vi "DS402-manager-Main.vi"() -> ()   [LabVIEW 2016]
uses:
  NationalInstruments.VeriStand.SystemStorageUI
  NationalInstruments.VeriStand.SystemStorage
  <vilib>/NI Veristand/Templates/Workspace Tool Support/Workspace Tool Message Bus.ctl
  <vilib>/NI Veristand/Templates/Workspace Tool Support/Workspace Tool Message (String).ctl
  <vilib>/NI Veristand/Templates/Workspace Tool Support/Workspace Tool Response (String).ctl
  <vilib>/NI Veristand/Templates/Workspace Tool Support/Workspace Tool Message (Byte Array).ctl
  <vilib>/NI Veristand/Templates/Workspace Tool Support/Workspace Tool Response (Byte Array).ctl
  _qmh/controls/UI Data.ctl
  _qmh/support/Message Queue/Enqueue Message (Single).vi
  <vilib>/Utility/error.llb/Error Cluster From Error Code.vi
  <vilib>/NI Veristand/Execution/Workspace/NI VeriStand - Get Multiple Channel Values.vi
  <vilib>/ErrorRing/Error Ring.xnode
  <vilib>/NI VeriStand/Execution/Workspace/NI_VS Workspace ExecutionAPI.lvlib
  <vilib>/NI Veristand/UI Controls/System Definition Tree/NI_VS UI System Tree.lvlib
  ds402mgr_Helper/ds402mgr_Helper.lvlib
  _qmh/support/User Event - Stop/User Event - Stop.lvlib
  _qmh/support/Message Queue/Message Queue.lvlib
  <vilib>/NI VeriStand/Templates/Workspace Tool Support/NI VeriStand - Workspace Tool Support.lvlib
panel:
  in  "Targets":i32(listbox)
  out "Detected at":timestamp
  out "Error":bool
  out "Slave Transition State history":string
  out "Slave State - Current":string
  in  "Tab Control":enum32{"Debug", "SDO", "Slave Diagnostics"}(tab)
  out "names":string[](array[string])
  out "types":i32[](array[ring]) items=["K_STRING", "K_BOOL", "K_I32", "K_U32", "K_DOUBLE", "K_U64", "K_VARIANT", "K_DEPENDENTFILE", "K_DEPENDENTNODE", "K_DATASOURCENODE", "K_U16", "K_DBLARR", "K_U32ARR", "K_I32ARR", "K_STRINGARR", "K_DICTIONARY", "K_DICTIONARYARR", "K_BINARYSTRING", "K_I16", "K_I64", "K_BOOLARR", "K_U64ARR", "K_U16ARR", "K_I64ARR", "K_I16ARR"]
  in  "width":enum16{"U8", "U16", "U32"}(ring)
  in  "Value to Write":i32
  out "Value Read":i32
  in  "Blocking Write":bool=TRUE
  in  "Abort Write":bool
  in  "Do Action":bool
  in  "Action":enum16{"Read", "Write"}(ring)
  out "Raw Data Read":u8[](array[numeric]) format="%.0x"
  out "Raw  - Data to Write":u8[](array[numeric]) format="%.0x"
  in  "Cleare Errors":bool
  out "Error Ext Para":i32[](array[numeric]) format="%.0x"
  out "Error Ext":u32
  out "Last Error":i32 format="%.0x"
  out "Abort Code":u32 format="%.0x"
  out "EMCY Data":T1 {"Error Code" format="%.0x"}
  out "Error Out":errorcluster
  in  "Action 4":bool
  in  "Action 3":bool
  in  "Action 2":bool
  in  "Action 1":bool
  out "Slave Information":string
  in  "NIVS.Message Bus":T2
  in  "Stop":bool
  in  "NIVS.System Definition Root":refnum<k24>
  in  "Select EtherCAT Slave":refnum<k24>(container)
  in  "NIVS.Project File Path":path
  in  "NIVS.Workspace Event":refnum<event-registration>
  out "System Times":dbl[](array[numeric]) format="%<%H:%M:%S%3u>t"
  out "Targets":string[](array[string])
  in  "NIVS.Gateway IP Address":string
  in  "NIVS.INI File Path":path
  # "With the assistance of the NI VeriStand Execution API, a tool has access to streaming data running on the target."
  # "This is the file path to the VeriStand system definition file. You can read or write to the file using the System Definition API."
  # "This is the root reference to the active System Definition file. You could use this to read the configuration or populate a tree with channels. You are free to close this reference, but it will be closed for you if you don't."
  # "This is the IP Address of the VeriStand Gateway to which the Workspace is connected. Use this to open all the .NET Manager references. Usually the Gateway is running on localhost, but it could be running on a neighbor's machine."
  # "This registered string User Event is used to help instruct your tool to shut down when the Workspace is closing."
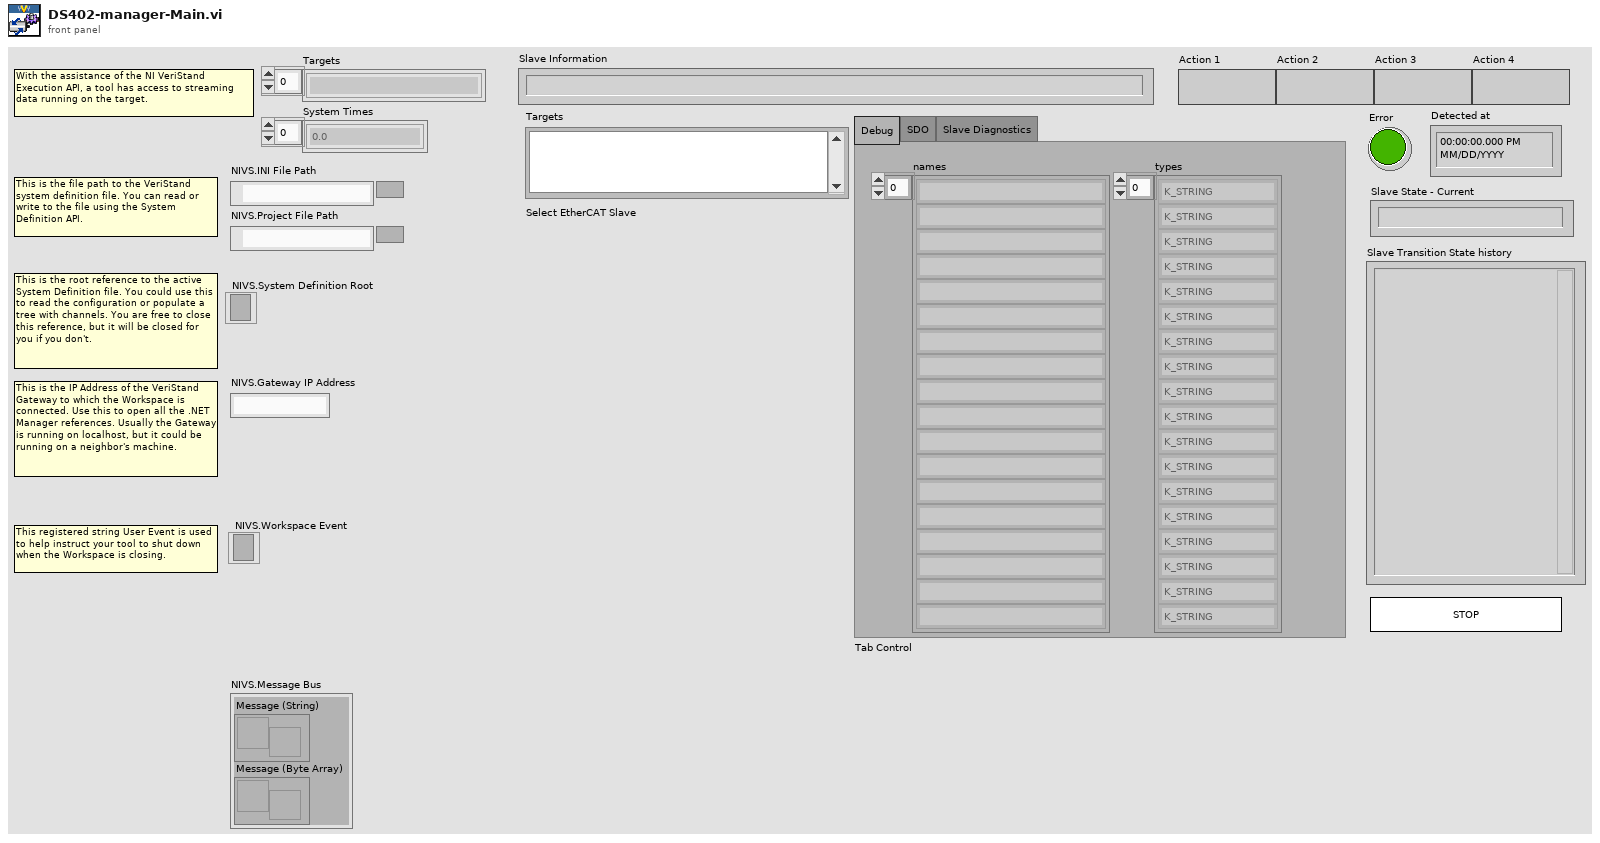
[diagram p1: front panel]
types:
  T1 = cluster{"Emergency Data":dbl[], "Error Register":u8, "Error Code":u16}
  T2 = typedef "NI VeriStand - Workspace Tool Support.lvlib/Workspace Tool Message Bus.ctl" = cluster{"Message (String)":refnum<user-event>, "Message (Byte Array)":refnum<user-event>}
  T3 = typedef "UI Data.ctl" = cluster{"Boolean <Replace Me>":bool, "String <Replace Me>":string, "Numeric <Replace Me>":dbl, "Do Something Ref":refnum<vi>, "Do Something Else Ref":refnum<vi>, "Data Display Ref":refnum<vi>, "Exit Button Ref":refnum<vi>}
  T4 = typedef "NI_VS Workspace ExecutionAPI.lvlib/WorkspaceAPI.ctl" = refnum<k24>
  T5 = typedef "ds402mgr_Helper.lvlib/_targetDetails.ctl" = cluster{"IP address":string, "NodeRef":refnum<k24>}
  T6 = typedef "NI_VS UI System Tree.lvlib/Callback Type.ctl" = cluster{"Net Callbacks":refnum<k27>[], "Event":T7}
  T7 = typedef "NI_VS UI System Tree.lvlib/Net Event Data Ref.ctl" = refnum<user-event>
  T8 = typedef "Message Queue.lvlib/All Message Queues.ctl" = cluster{"UI":refnum<queue>}
  T9 = typedef "NI_VS Workspace ExecutionAPI.lvlib/SystemStateEventRef.ctl" = cluster{"CustDatRef":refnum<user-event>, "EvtRef":refnum<k27>, "Target State User Event":refnum<user-event>}
  T10 = typedef "NI_VS Workspace ExecutionAPI.lvlib/SystemStateRegEventRef.ctl" = refnum<event-registration>
  T11 = cluster{"Event Registration Refnum":refnum<event-registration>, "NIVS.Workspace Event":refnum<event-registration>, "SystemChangeEventRef":T10}
  T12 = typedef "NI_VS UI System Tree.lvlib/Node Ref.ctl" = refnum<k24>
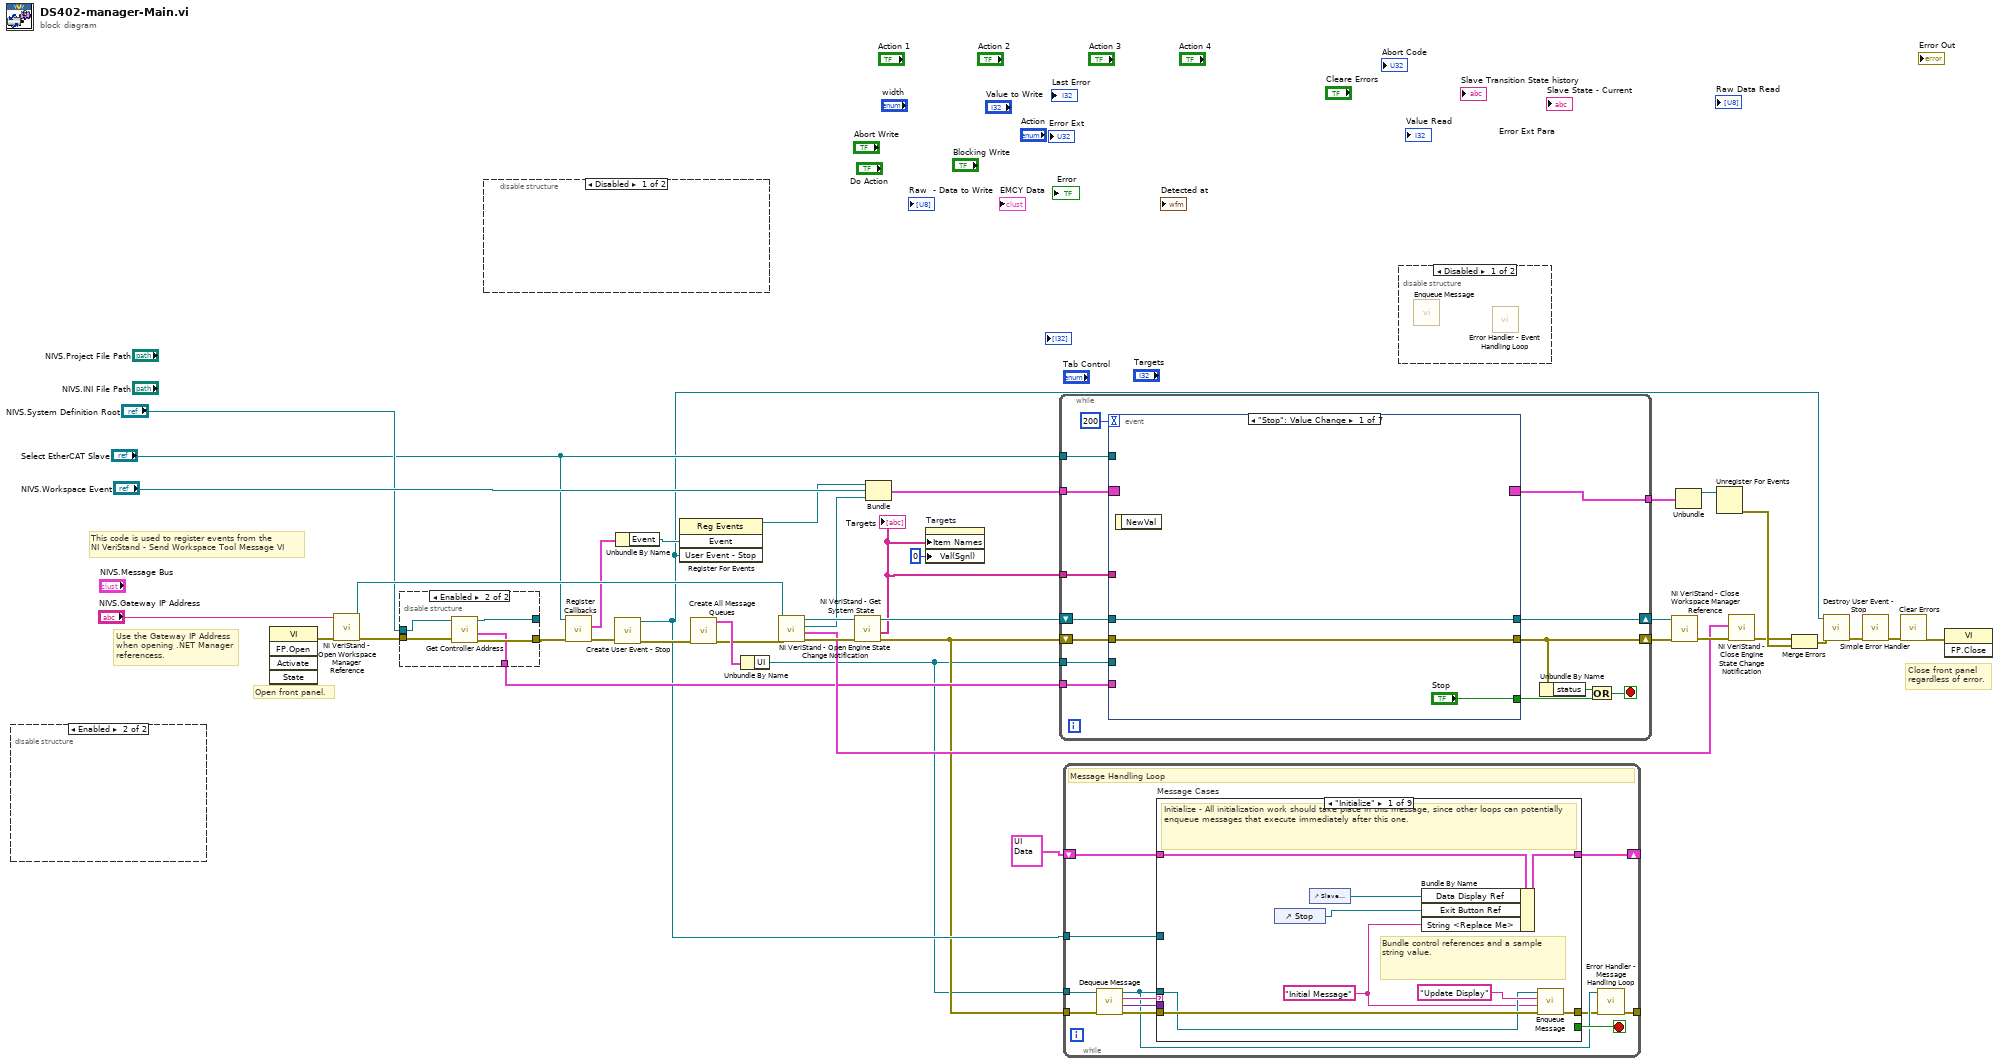
[diagram p0: block diagram]
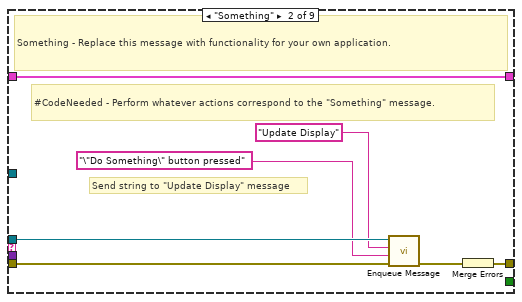
[diagram p3: hidden frame]
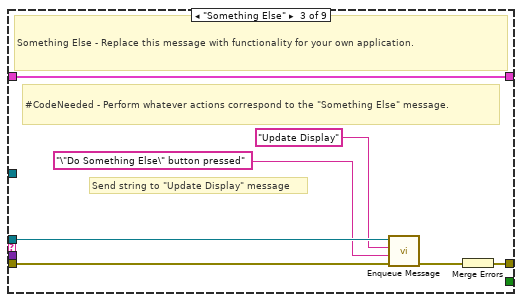
[diagram p4: hidden frame]
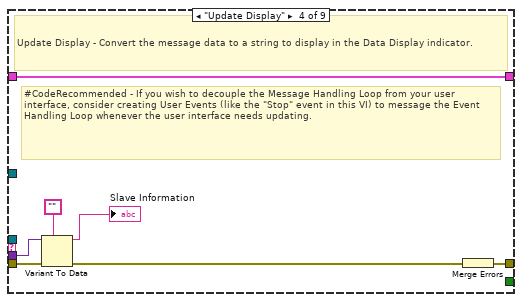
[diagram p5: hidden frame]
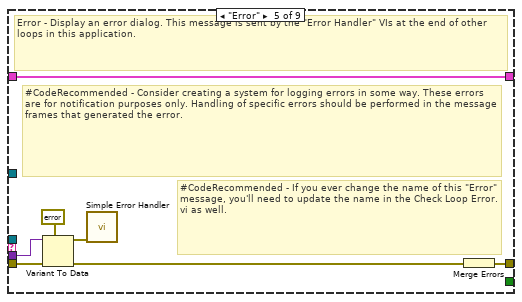
[diagram p6: hidden frame]
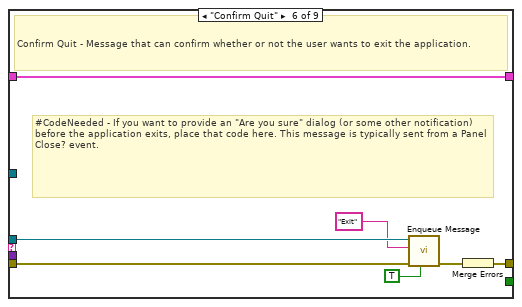
[diagram p7: hidden frame]
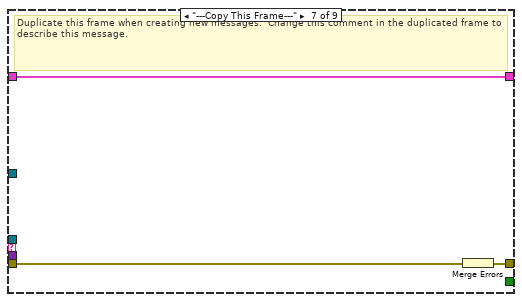
[diagram p8: hidden frame]
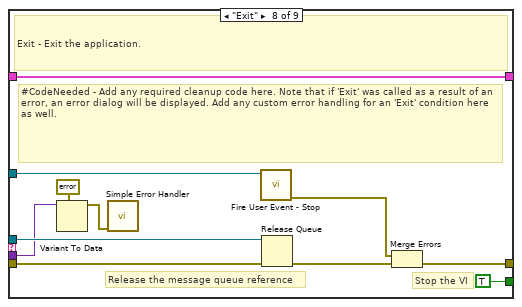
[diagram p9: hidden frame]
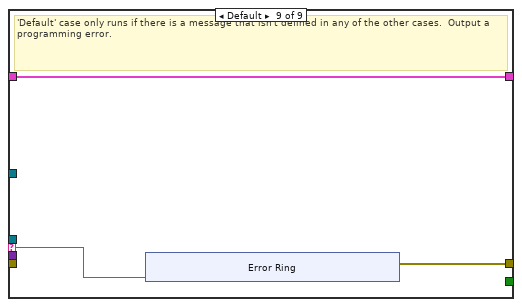
[diagram p10: hidden frame]
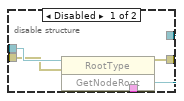
[diagram p12: hidden frame]
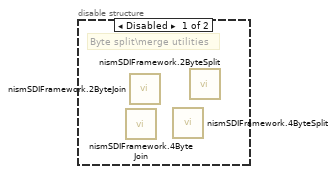
[diagram p13: hidden frame]
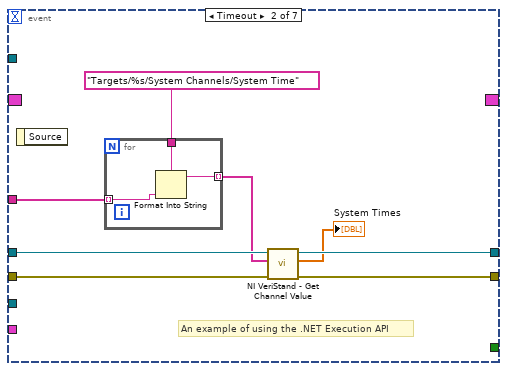
[diagram p14: hidden frame]
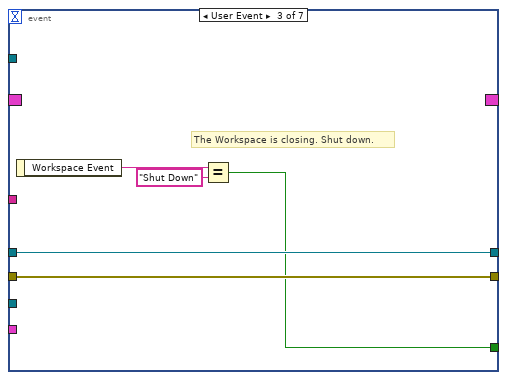
[diagram p15: hidden frame]
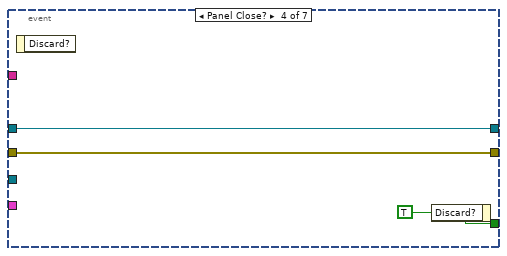
[diagram p16: hidden frame]
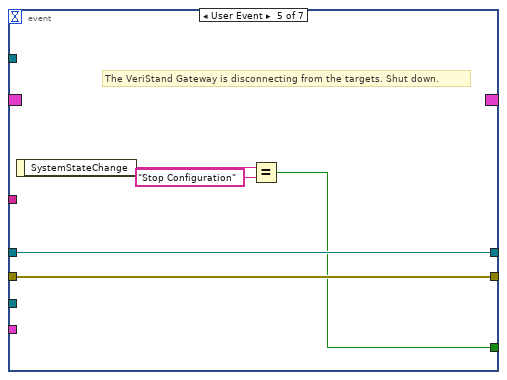
[diagram p17: hidden frame]
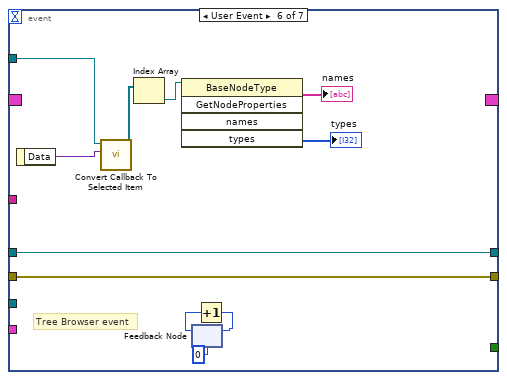
[diagram p18: hidden frame]
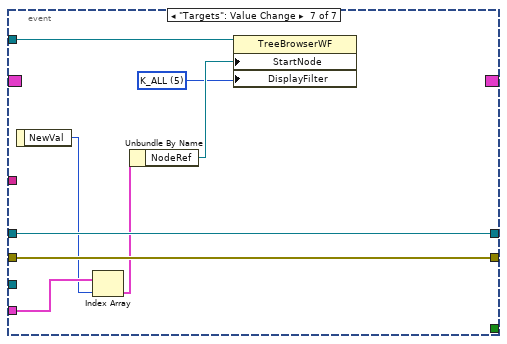
[diagram p19: hidden frame]
diagram:
  # "This code is used to register events from the\nNI VeriStand - Send Workspace Tool Message VI"
  # "Use the Gateway IP Address when opening .NET Manager referencess."
  # "Close front panel\nregardless of error."
  # "Open front panel."
  n1 = disable-structure shown="Enabled" {
    frame Disabled {
      # "Byte split\\merge utilities"
      n2 = call <vilib>:"nismSDIFramework.4ByteJoin.vi"() -> ()  [unwired: 11 in, 1 out]
      n3 = call <vilib>:"nismSDIFramework.2ByteJoin.vi"() -> ()  [unwired: 11 in, 1 out]
      n4 = call <vilib>:"nismSDIFramework.4ByteSplit.vi"() -> ()  [unwired: 8 in, 4 out]
      n5 = call <vilib>:"nismSDIFramework.2ByteSplit.vi"() -> ()  [unwired: 10 in, 2 out]
    }
    frame Enabled {
    }
  }
  n6 = invoke class="VI" method="FP.Open"() -> (error out=w26:errorcluster)  [unwired: 5 in, 4 out]
  n7 = call <vilib>:"NI VeriStand - Open Workspace Manager Reference.vi"("error in (no error)"=w26, "Gateway IP Address (\"\": localhost)"="NIVS.Gateway IP Address") -> ("error out"=w17:errorcluster, "WorkspaceManager"=w34:T4)  [unwired: 8 in]
  n8 = disable-structure shown="Enabled" {
    disable-tunnel: [w43 w46] -> _
    disable-tunnel: [w42 w47] -> w16
    disable-tunnel: "NIVS.System Definition Root" -> [w41 w48]
    disable-tunnel: w17 -> [w40 w45]
    disable-tunnel: [_ w44] -> w15
    frame Disabled {
      n9 = invoke class="RootType" method="GetNodeRoot"(reference=w41, error in=w40) -> (error out=w42:errorcluster, "GetNodeRoot"=w43:refnum<k24>)  [unwired: 1 in, 1 out]
    }
    frame Enabled {
      n10 = call "Get Controller Address.vi"("error in (no error)"=w45, "NIVS.System Definition Root In"=w48) -> ("error out"=w47:errorcluster, "Results"=w44:T5[], "NIVS.System Definition Root Out"=w46:refnum<k24>)  [unwired: 5 in, 2 out]
    }
  }
  n11 = disable-structure shown="Disabled" {
    frame Disabled {
    }
    frame Enabled {
    }
  }
  n12 = call <vilib>:"Register Callbacks.vi"("error in (no error)"=w16, "System Definition Tree"="Select EtherCAT Slave") -> ("error out"=w12:errorcluster, "Callbacks"=w20:T6)  [unwired: 7 in, 1 out]
  n13 = call "Create User Event - Stop.vi"("error in (no error)"=w12) -> ("error out"=w10:errorcluster, "User Event - Stop"=w3:refnum<user-event>)  [unwired: 9 in]
  n14 = Unbundle By Name(w20) -> ("Event"=w19:T7)
  n15 = register-events(w19, w3) -> (reference out=w18:refnum<event-registration>)  [unwired: 2 in, 1 out]
  n16 = call "Create All Message Queues.vi"("error in (no error)"=w10) -> ("error out"=w9:errorcluster, "Message Queues out"=w11:T8)  [unwired: 9 in]
  n17 = Unbundle By Name(w11) -> ("UI"=w1:refnum<queue>)
  n18 = call <vilib>:"NI VeriStand - Open Engine State Change Notification.vi"("error in (no error)"=w9, "WorkspaceManager in"=w34) -> ("error out"=w38:errorcluster, "SystemStateRefs"=w29:T9, "SystemChangeEventRef"=w23:T10, "WorkspaceManager out"=w39:T4)  [unwired: 6 in]
  n19 = call <vilib>:"NI VeriStand - Get System State.vi"("error in (no error)"=w38, "WorkspaceManager in"=w39) -> ("error out"=w2:errorcluster, "Targets"=w14:string[], "WorkspaceManager  out"=w28:T4)  [unwired: 5 in, 2 out]
  "Targets" <- w14
  n20 = Bundle("Event Registration Refnum"=w18, "NIVS.Workspace Event"="NIVS.Workspace Event", "SystemChangeEventRef"=w23) -> (w33:T11)  [unwired: 1 in]
  n21 = property on="Targets" class="LstBox (strict)"("Item Names"=w14, "Val(Sgnl)"=0 ("Value (Signaling)")) -> ()  [unwired: 2 in, 2 out]
  n22 = while {
    tunnel: w33 -> [w62]
    tunnel: [w61] -> w32
    shift-right: [w55] -> w35
    shift-left: w2 -> [w59]
    shift-right: [w58] -> w36
    shift-left: w28 -> [w60]
    tunnel: "Select EtherCAT Slave" -> [w52]
    tunnel: w15 -> [w51]
    tunnel: w14 -> [w50]
    tunnel: w1 -> [w49]
    stop <- w53 stop-if-true
    n23 = event shown="[0] \"Stop\": Value Change" {
      selector: w62 -> [_ _ _ _ _ _ _]
      dyn-events: [_ _ _ _ _ _ _] -> w61
      timeout: 200 -> [_ _ _ _ _ _ _]
      tunnel: ["Stop" _ w77 w82 w85 _ _] -> w54
      tunnel: w60 -> [w64 w73 w80 w83 w88 w99 w107]
      tunnel: w59 -> [w65 w72 w81 w84 w89 w100 w108]
      tunnel: [w65 w68 w81 w84 w89 w100 w108] -> w55
      tunnel: [w64 w69 w80 w83 w88 w99 w107] -> w58
      tunnel: w52 -> [_ _ _ _ _ w95 w104]
      tunnel: w51 -> [_ _ _ _ _ _ w106]
      tunnel: w50 -> [_ w66 _ _ _ _ _]
      tunnel: w49 -> [_ _ _ _ _ _ _]
      event "Stop": Value Change {
        n24 = event-data() -> ()  [unwired: 1 in, 1 out]
      }
      event Timeout {
        # "An example of using the .NET Execution API"
        n25 = event-data() -> ()  [unwired: 1 in, 1 out]
        n26 = for {
          tunnel: "Targets/%s/System Channels/System Time" ("format string") -> [w76]
          tunnel: [w75] -> w70 mode=indexing
          tunnel: w66 -> [w74] mode=indexing
          n27 = Format Into String(format string=w76, w74) -> (resulting string=w75:string)  [unwired: 2 in, 1 out]
        }
        n28 = call-poly <vilib>:"NI VeriStand - Get Channel Value.vi"("error in (no error)"=w72, "Channels"=w70, "WorkspaceManager in"=w73) -> ("error out"=w68:errorcluster, "Values"=→"System Times":dbl[], "WorkspaceManager out"=w69:T4)  [unwired: 6 in]
      }
      event User Event {
        # "The Workspace is closing. Shut down."
        n29 = event-data() -> ("Workspace Event"=w79:string)  [unwired: 1 in]
        n30 = Equal?(x=w79, y="Shut Down") -> (x = y?=w77:bool)
      }
      event Panel Close? {
        w82 = TRUE ("Discard?")
        n31 = event-data() -> ()  [unwired: 1 in, 1 out]
        n32 = event-data("Discard?"=w82) -> ()  [unwired: 1 in, 1 out]
      }
      event User Event {
        # "The VeriStand Gateway is disconnecting from the targets. Shut down."
        n33 = event-data() -> ("SystemStateChange"=w87:string)  [unwired: 1 in]
        n34 = Equal?(x=w87, y="Stop Configuration") -> (x = y?=w85:bool)
      }
      event User Event {
        # "Tree Browser event"
        n35 = event-data() -> ("Data"=w96:variant)  [unwired: 1 in]
        n36 = call <vilib>:"Convert Callback To Selected Item.vi"("Data"=w96, "SystemDefinitionBrowser Ref"=w95) -> ("Selected Item"=w93:T12[])  [unwired: 8 in, 1 out]
        n37 = Index Array(array=w93) -> (element=w91:T12)  [unwired: 1 in]
        n38 = invoke class="BaseNodeType" method="GetNodeProperties"(reference=w91) -> ("names"=→"names":string[], "types"=→"types":i32[])  [unwired: 4 in, 3 out]
        n39 = feedback #1(0) -> (w90:i32)
        n40 = Increment(x=w90) -> (x+1=w98:i32)
        n41 = feedback-in #1(w98) -> ()
      }
      event "Targets": Value Change {
        w101 = u8 5 items=["K_CHAN_R", "K_CHAN_W", "K_CHAN_RW", "K_CHAN_VOLT", "K_CHAN_FAULT", "K_ALL", "K_CUSTOM", "K_CHAN_R_VIS", "K_CHAN_W_VIS", "K_CHAN_RW_VIS", "K_CHAN_VOLT_VIS", "K_CHAN_FAULT_VIS"] ("DisplayFilter")
        n42 = event-data() -> ("NewVal"=w105:i32)  [unwired: 1 in]
        n43 = Index Array(array=w106, index=w105) -> (element=w103:T5)
        n44 = Unbundle By Name(w103) -> ("NodeRef"=w102:refnum<k24>)
        n45 = property class="TreeBrowserWF"(reference=w104, "StartNode"=w102, "DisplayFilter"=w101) -> ()  [unwired: 1 in, 2 out]
      }
    }
    n46 = Unbundle By Name(w55) -> ("status"=w56:bool)
    n47 = Compound Arithmetic op=OR(w56, w54) -> (w53:bool)
  }
  n48 = while {
    tunnel: w1 -> [w112]
    shift-right: [w119] -> _
    shift-left: T3 {"Boolean <Replace Me>"=FALSE, "String <Replace Me>"="", "Numeric <Replace Me>"=0.0, "Do Something Ref"=refnum, "Do Something Else Ref"=refnum, "Data Display Ref"=refnum, "Exit Button Ref"=refnum} ("Data Cluster") -> [w120]
    tunnel: w3 -> [w117]
    tunnel: w2 -> [w116]
    tunnel: [w110] -> _
    stop <- w118 stop-if-true
    # "Message Handling Loop"
    n49 = call "Dequeue Message.vi"("error in (no error)"=w116, "Message Queue"=w112) -> ("error out"=w115:errorcluster, "Message Data"=w113:variant, "Message"=w114:string, "dup Message Queue"=w111:refnum<queue>)  [unwired: 6 in]
    n50 = case "Message Cases" shown="\"Initialize\"" w114 {
      selector: w114 -> [_ _ _ _ _ _ _ _ w179]
      tunnel: w111 -> [w124 w132 w139 _ _ w160 _ w178 _]
      tunnel: w115 -> [w128 w134 w141 w148 w157 w164 w167 w171 _]
      tunnel: [w129 w135 w142 w149 w151 w162 w165 w174 w180] -> w109
      tunnel: w120 -> [w127 w136 w143 w150 w156 w163 w166 w177 w181]
      tunnel: [w126 w136 w143 w150 w156 w163 w166 w177 w181] -> w119
      tunnel: [_ _ _ _ _ _ _ TRUE _] -> w118
      tunnel: w113 -> [_ _ _ w147 w155 _ _ w168 _]
      tunnel: w117 -> [_ _ _ _ _ _ _ w173 _]
      frame "Initialize" {
        w123 = "Initial Message" ("Initial Message")
        # "Bundle control references and a sample string value."
        # "Initialize - All initialization work should take place in this message, since other loops can potentially enqueue messages that execute immediately after this one."
        n51 = control-ref of="Stop"() -> (w121:refnum<vi>)
        n52 = control-ref of="Slave Information"() -> (w122:refnum<vi>)
        n53 = Bundle By Name(cluster=w127, "Data Display Ref"=w122, "Exit Button Ref"=w121, "String <Replace Me>"=w123) -> (w126:T3)
        n54 = call-poly "Enqueue Message.vi"("error in (no error)"=w128, "Message Data"=w123, "Message"="Update Display", "Message Queue"=w124) -> ("error out"=w129:errorcluster)  [unwired: 6 in, 1 out]
      }
      frame "Something" {
        # "Send string to \"Update Display\" message"
        # "#CodeNeeded - Perform whatever actions correspond to the \"Something\" message."
        # "Something - Replace this message with functionality for your own application."
        n55 = call-poly "Enqueue Message.vi"("error in (no error)"=w134, "Message Data"="\"Do Something\" button pressed" ("\"Do Something\" button pressed"), "Message"="Update Display", "Message Queue"=w132) -> ("error out"=w133:errorcluster)  [unwired: 6 in, 1 out]
        n56 = Merge Errors(w133) -> (w135:errorcluster)
      }
      frame "Something Else" {
        # "Send string to \"Update Display\" message"
        # "#CodeNeeded - Perform whatever actions correspond to the \"Something Else\" message."
        # "Something Else - Replace this message with functionality for your own application."
        n57 = call-poly "Enqueue Message.vi"("error in (no error)"=w141, "Message Data"="\"Do Something Else\" button pressed" ("\"Do Something Else\" button pressed"), "Message"="Update Display", "Message Queue"=w139) -> ("error out"=w140:errorcluster)  [unwired: 6 in, 1 out]
        n58 = Merge Errors(w140) -> (w142:errorcluster)
      }
      frame "Update Display" {
        # "#CodeRecommended - If you wish to decouple the Message Handling Loop from your user interface, consider creating User Events (like the \"Stop\" event in this VI) to message the Event Handling Loop whenever the user interface needs updating."
        # "Update Display - Convert the message data to a string to display in the Data Display indicator."
        n59 = Variant To Data(error in=w148, type="", Variant=w147) -> (data=→"Slave Information":string, error out=w145:errorcluster)
        n60 = Merge Errors(w145) -> (w149:errorcluster)
      }
      frame "Error" {
        # "#CodeRecommended - If you ever change the name of this \"Error\" message, you'll need to update the name in the Check Loop Error.vi as well."
        # "#CodeRecommended - Consider creating a system for logging errors in some way. These errors are for notification purposes only. Handling of specific errors should be performed in the message frames that generated the error."
        # "Error - Display an error dialog. This message is sent by the \"Error Handler\" VIs at the end of other loops in this application."
        n61 = Variant To Data(error in=w157, type=errorcluster {"status"=FALSE, "code"=0, "source"=""} ("error constant"), Variant=w155) -> (data=w153:errorcluster, error out=w152:errorcluster)
        n62 = call <vilib>:"Simple Error Handler.vi"("error in (no error)"=w153) -> ()  [unwired: 4 in, 5 out]
        n63 = Merge Errors(w152) -> (w151:errorcluster)
      }
      frame "Confirm Quit" {
        # "#CodeNeeded - If you want to provide an \"Are you sure\" dialog (or some other notification) before the application exits, place that code here. This message is typically sent from a Panel Close? event."
        # "Confirm Quit - Message that can confirm whether or not the user wants to exit the application."
        n64 = call-poly "Enqueue Message.vi"("Priority Message? (F)"=TRUE, "error in (no error)"=w164, "Message"="Exit", "Message Queue"=w160) -> ("error out"=w161:errorcluster)  [unwired: 6 in, 1 out]
        n65 = Merge Errors(w161) -> (w162:errorcluster)
      }
      frame "---Copy This Frame---" {
        # "Duplicate this frame when creating new messages.  Change this comment in the duplicated frame to describe this message."
        n66 = Merge Errors(w167) -> (w165:errorcluster)
      }
      frame "Exit" {
        # "Stop the VI"
        # "Release the message queue reference"
        # "#CodeNeeded - Add any required cleanup code here. Note that if 'Exit' was called as a result of an error, an error dialog will be displayed. Add any custom error handling for an 'Exit' condition here as well."
        # "Exit - Exit the application."
        n67 = Variant To Data(type=errorcluster {"status"=FALSE, "code"=0, "source"=""} ("error constant"), Variant=w168) -> (data=w169:errorcluster)  [unwired: 1 in, 1 out]
        n68 = call <vilib>:"Simple Error Handler.vi"("error in (no error)"=w169) -> ()  [unwired: 4 in, 5 out]
        n69 = call "Fire User Event - Stop.vi"("User Event - Stop"=w173) -> ("error out"=w172:errorcluster)  [unwired: 10 in]
        n70 = Release Queue(queue=w178, error in (no error)=w171) -> (error out=w175:errorcluster)  [unwired: 1 in, 2 out]
        n71 = Merge Errors(w172, w175) -> (w174:errorcluster)
      }
      frame Default {
        # "'Default' case only runs if there is a message that isn't defined in any of the other cases.  Output a programming error."
        n72 = xnode "Error Ring"("parameter 0"=w179) -> ("error out"=w180:errorcluster)
      }
    }
    n73 = call "Error Handler - Message Handling Loop.vi"("error in (no error)"=w109, "Message Queue"=w111) -> ("dup error in"=w110:errorcluster)  [unwired: 8 in, 1 out]
  }
  n74 = disable-structure shown="Disabled" {
    frame Disabled {
      n75 = call-poly "Enqueue Message.vi"() -> ()  [unwired: 10 in, 2 out]
      n76 = call "Error Handler - Event Handling Loop.vi"() -> ()  [unwired: 10 in, 2 out]
    }
    frame Enabled {
    }
  }
  n77 = call <vilib>:"NI VeriStand - Close Workspace Manager Reference.vi"("error in (no error)"=w35, "WorkspaceManager"=w36) -> ("error out"=w30:errorcluster)  [unwired: 9 in]
  n78 = Unbundle(w32) -> ("Event Registration Refnum"=w31:refnum<event-registration>)  [unwired: 2 out]
  n79 = Unregister For Events(event registration refnum=w31) -> (error out=w6:errorcluster)  [unwired: 1 in]
  n80 = call <vilib>:"NI VeriStand - Close Engine State Change Notification.vi"("error in (no error)"=w30, "SystemStateRefs"=w29) -> ("error out"=w5:errorcluster)  [unwired: 9 in]
  n81 = Merge Errors(w5, w6) -> (w7:errorcluster)
  n82 = call "Destroy User Event - Stop.vi"("error in (no error)"=w7, "User Event - Stop"=w3) -> ("error out"=w4:errorcluster)  [unwired: 9 in]
  n83 = call <vilib>:"Simple Error Handler.vi"("error in (no error)"=w4) -> ("error out"=w25:errorcluster)  [unwired: 4 in, 4 out]
  n84 = call <vilib>:"Clear Errors.vi"("error in (no error)"=w25) -> ("error out"=w24:errorcluster)  [unwired: 5 in, 1 out]
  n85 = invoke class="VI" method="FP.Close"(error in=w24) -> ()  [unwired: 2 in, 3 out]
